vi "Aging Run.vi"(8 "UDL":path, 9 "error in":errorcluster, 10 "Arduino":refnum<visa-resource-name>, 11 "System Number":string) -> (1 "error out":errorcluster, 2 "Arduino":refnum<visa-resource-name>)   [LabVIEW 2024]
uses:
  <vilib>/addons/database/Connection.llb/DB Tools Open Connec (Path).vi
  <vilib>/addons/database/_DB Variant To Data/Database Variant To Data.xnode
  <vilib>/addons/database/NI_Database_API.lvlib
panel:
  out "Commands":string[](array[string])
  out "IsSine":bool=TRUE
  out "Frequency":string
  out "DC_SN":string
  out "Nominal Frequency":string
  out "OscVoltage":string
  out "TimeStart":string
  out "Current Position":i8
  out "Current Rack":i8
types:
  T1 = typedef "NI_Database_API.lvlib/Conn ObjectReference.ctl" = refnum<k1>
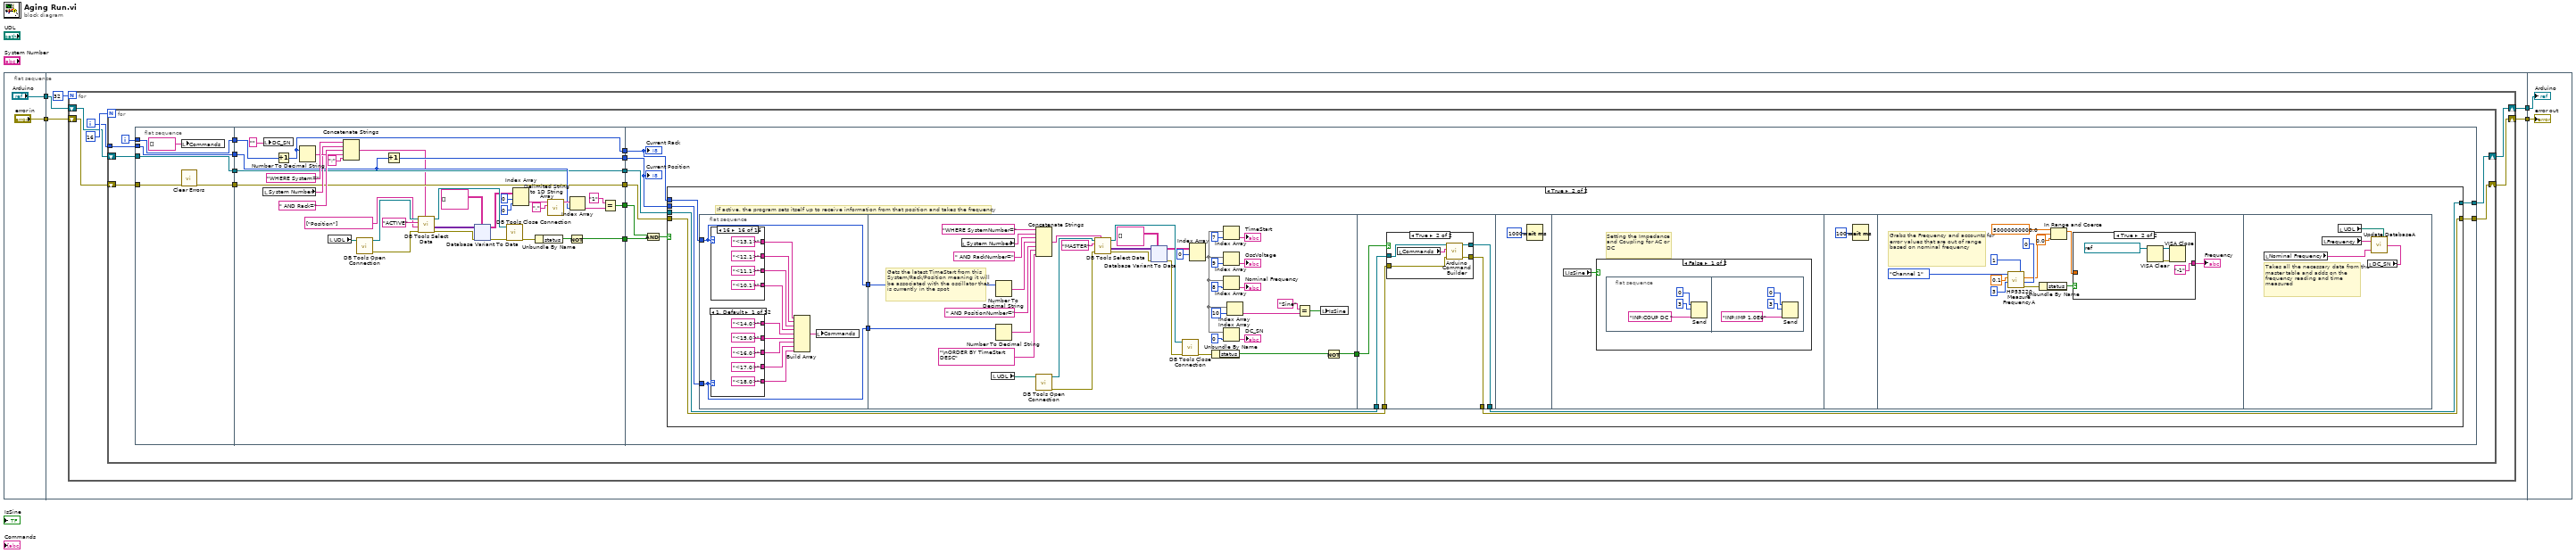
[diagram p0: block diagram]
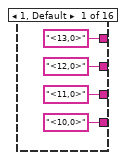
[diagram p3: hidden frame]
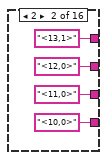
[diagram p4: hidden frame]
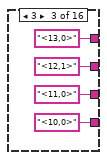
[diagram p5: hidden frame]
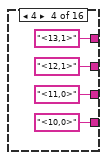
[diagram p6: hidden frame]
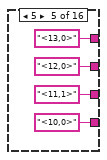
[diagram p7: hidden frame]
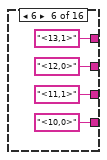
[diagram p8: hidden frame]
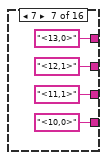
[diagram p9: hidden frame]
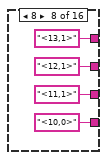
[diagram p10: hidden frame]
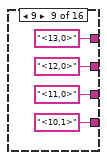
[diagram p11: hidden frame]
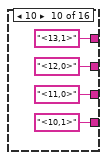
[diagram p12: hidden frame]
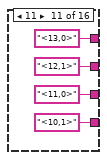
[diagram p13: hidden frame]
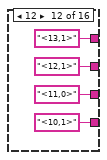
[diagram p14: hidden frame]
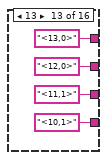
[diagram p15: hidden frame]
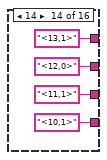
[diagram p16: hidden frame]
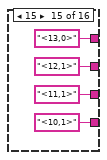
[diagram p17: hidden frame]
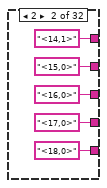
[diagram p18: hidden frame]
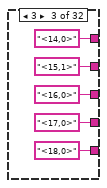
[diagram p19: hidden frame]
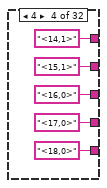
[diagram p20: hidden frame]
diagram:
  n1 = flat-sequence {
    tunnel: ["Arduino"] -> w2
    tunnel: ["error in"] -> w1
    tunnel: [w10] -> w4
    tunnel: [w9] -> w3
    tunnel: w2 -> [w8]
    tunnel: w1 -> [w7]
    tunnel: w4 -> [w507]
    tunnel: w3 -> [w506]
    frame #0 {
    }
    frame #1 {
      n2 = for {
        N: 32 -> [_]
        shift-right: [w15] -> w10
        shift-left: w8 -> [w13]
        shift-right: [w14] -> w9
        shift-left: w7 -> [w12]
        i -> [w16]
        n3 = for {
          N: 16 -> [_]
          tunnel: w16 -> [w31]
          shift-right: [w33] -> w14
          shift-left: w12 -> [w24]
          shift-right: [w32] -> w15
          shift-left: w13 -> [w23]
          i -> [w30]
          n4 = flat-sequence {
            tunnel: w30 -> [w38]
            tunnel: w31 -> [w39]
            tunnel: [w39] -> w26
            tunnel: [w38] -> w25
            tunnel: w24 -> [w37]
            tunnel: w23 -> [w35]
            tunnel: [w35] -> w20
            tunnel: [w34] -> w18
            tunnel: [w59] -> w29
            tunnel: [w58] -> w28
            tunnel: [w57] -> w27
            tunnel: w26 -> [w61]
            tunnel: w25 -> [w60]
            tunnel: [w55] -> w22
            tunnel: [w54] -> w21
            tunnel: w20 -> [w54]
            tunnel: [w53] -> w19
            tunnel: w18 -> [w53]
            tunnel: [w127] -> w33
            tunnel: [w126] -> w32
            tunnel: w29 -> [w123]
            tunnel: w28 -> [w124]
            tunnel: w27 -> [w125]
            tunnel: w22 -> [w122]
            tunnel: w21 -> [w120]
            tunnel: w19 -> [w119]
            frame #0 {
              n5 = local write "Commands"(string[] [] ("Commands")) -> ()
              n6 = call <vilib>:"Clear Errors.vi"("error in (no error)"=w37) -> ("error out"=w34:errorcluster)  [unwired: 5 in, 1 out]
            }
            frame #1 {
              n7 = local read "System Number"() -> (w70:string)
              n8 = local write "DC_SN"("" ("DC.SN")) -> ()
              n9 = Increment(x=w60) -> (x+1=w58:i32)
              n10 = Number To Decimal String(number=w58) -> (decimal integer string=w71:string)  [unwired: 1 in]
              n11 = local read "UDL"() -> (w44:path)
              n12 = Concatenate Strings("WHERE System=" ("SQL Query"), w70, " AND Rack=", w71, ";" ("string")) -> (w46:string)
              n13 = call-poly <vilib>:"DB Tools Open Connection.vi"("connection information"=w44) -> ("error out"=w50:errorcluster, "connection reference"=w51:T1)  [unwired: 7 in]
              n14 = Increment(x=w61) -> (x+1=w57:i32)
              n15 = call <vilib>:"DB Tools Select Data.vi"("condition"=w46, "error in (no error)"=w50, "columns"=string[] ["Position"], "table"="ACTIVE", "connection reference"=w51) -> ("error out"=w43:errorcluster, "data"=w48:variant[][], "connection reference out"=w52:T1)  [unwired: 1 in]
              n16 = xnode "Database Variant To Data"("database variant"=w48, "error in (no error)"=w43, "type"=string[][] [] ("table")) -> ("data"=w45:string[][], "error out"=w41:errorcluster)
              n17 = call <vilib>:"DB Tools Close Connection.vi"("error in (no error)"=w41, "connection reference"=w52) -> ("error out"=w42:errorcluster)  [unwired: 5 in]
              n18 = Index Array(array=w45, index (row)=0 ("disabled index (row)"), index (col)=0 ("disabled index (col)")) -> (element=w69:string)
              n19 = Unbundle By Name(w42) -> ("status"=w56:bool)
              n20 = call <vilib>:"Delimited String to 1D String Array.vi"("delimiter"=",", "delimited string"=w69) -> ("string array"=w66:string[])  [unwired: 9 in]
              n21 = Not(x=w56) -> (.not. x?=w55:bool)
              n22 = Index Array(array=w66, index=w61) -> (element=w65:string)
              n23 = Equal?(x="1", y=w65) -> (x = y?=w59:bool)
            }
            frame #2 {
              n24 = And(x=w123, y=w122) -> (x .and. y?=w121:bool)
              n25 = case shown="True" w121 {
                tunnel: w125 -> [_ w138]
                tunnel: w124 -> [_ w137]
                tunnel: [w128 w136] -> w127
                tunnel: [w129 w135] -> w126
                tunnel: w119 -> [w128 w134]
                tunnel: w120 -> [w129 w133]
                frame False {
                  # "If inactive, nothing happens"
                }
                frame True {
                  # "If active, the program sets itself up to receive information from that position and takes the frequency"
                  n26 = flat-sequence {
                    tunnel: [w150] -> w132
                    tunnel: [w149] -> w131
                    tunnel: w137 -> [w149]
                    tunnel: w138 -> [w150]
                    tunnel: w131 -> [w402]
                    tunnel: w132 -> [w404]
                    tunnel: [w387] -> w130
                    tunnel: [w460] -> w136
                    tunnel: [w459] -> w135
                    tunnel: w134 -> [w458]
                    tunnel: w133 -> [w457]
                    tunnel: w130 -> [w456]
                    frame #0 {
                      n27 = case shown="16" w149 {
                        tunnel: ["<10,0>" ("string") "<10,0>" ("string") "<10,0>" ("string") "<10,0>" ("string") "<10,0>" ("string") "<10,0>" ("string") "<10,0>" ("string") "<10,0>" ("string") "<10,1>" ("string") "<10,1>" ("string") "<10,1>" ("string") "<10,1>" ("string") "<10,1>" ("string") "<10,1>" ("string") "<10,1>" ("string") "<10,1>" ("string")] -> w146
                        tunnel: ["<12,0>" ("string") "<12,0>" ("string") "<12,1>" ("string") "<12,1>" ("string") "<12,0>" ("string") "<12,0>" ("string") "<12,1>" ("string") "<12,1>" ("string") "<12,0>" ("string") "<12,0>" ("string") "<12,1>" ("string") "<12,1>" ("string") "<12,0>" ("string") "<12,0>" ("string") "<12,1>" ("string") "<12,1>" ("string")] -> w147
                        tunnel: ["<11,0>" ("string") "<11,0>" ("string") "<11,0>" ("string") "<11,0>" ("string") "<11,1>" ("string") "<11,1>" ("string") "<11,1>" ("string") "<11,1>" ("string") "<11,0>" ("string") "<11,0>" ("string") "<11,0>" ("string") "<11,0>" ("string") "<11,1>" ("string") "<11,1>" ("string") "<11,1>" ("string") "<11,1>" ("string")] -> w148
                        tunnel: ["<13,0>" ("string") "<13,1>" ("string") "<13,0>" ("string") "<13,1>" ("string") "<13,0>" ("string") "<13,1>" ("string") "<13,0>" ("string") "<13,1>" ("string") "<13,0>" ("string") "<13,1>" ("string") "<13,0>" ("string") "<13,1>" ("string") "<13,0>" ("string") "<13,1>" ("string") "<13,0>" ("string") "<13,1>" ("string")] -> w145
                        frame 1, Default {
                        }
                        frame 2 {
                        }
                        frame 3 {
                        }
                        frame 4 {
                        }
                        frame 5 {
                        }
                        frame 6 {
                        }
                        frame 7 {
                        }
                        frame 8 {
                        }
                        frame 9 {
                        }
                        frame 10 {
                        }
                        frame 11 {
                        }
                        frame 12 {
                        }
                        frame 13 {
                        }
                        frame 14 {
                        }
                        frame 15 {
                        }
                        frame 16 {
                        }
                      }
                      n28 = case shown="1, Default" w150 {
                        tunnel: ["<14,0>" ("string") "<14,1>" ("string") "<14,0>" ("string") "<14,1>" ("string") "<14,0>" ("string") "<14,1>" ("string") "<14,0>" ("string") "<14,1>" ("string") "<14,0>" ("string") "<14,1>" ("string") "<14,0>" ("string") "<14,1>" ("string") "<14,0>" ("string") "<14,1>" ("string") "<14,0>" ("string") "<14,1>" ("string") "<14,0>" ("string") "<14,1>" ("string") "<14,0>" ("string") "<14,1>" ("string") "<14,0>" ("string") "<14,1>" ("string") "<14,0>" ("string") "<14,1>" ("string") "<14,0>" ("string") "<14,1>" ("string") "<14,0>" ("string") "<14,1>" ("string") "<14,0>" ("string") "<14,1>" ("string") "<14,0>" ("string") "<14,1>" ("string")] -> w143
                        tunnel: ["<16,0>" ("string") "<16,0>" ("string") "<16,0>" ("string") "<16,0>" ("string") "<16,1>" ("string") "<16,1>" ("string") "<16,1>" ("string") "<16,1>" ("string") "<16,0>" ("string") "<16,0>" ("string") "<16,0>" ("string") "<16,0>" ("string") "<16,1>" ("string") "<16,1>" ("string") "<16,1>" ("string") "<16,1>" ("string") "<16,0>" ("string") "<16,0>" ("string") "<16,0>" ("string") "<16,0>" ("string") "<16,1>" ("string") "<16,1>" ("string") "<16,1>" ("string") "<16,1>" ("string") "<16,0>" ("string") "<16,0>" ("string") "<16,0>" ("string") "<16,0>" ("string") "<16,1>" ("string") "<16,1>" ("string") "<16,1>" ("string") "<16,1>" ("string")] -> w141
                        tunnel: ["<18,0>" ("string") "<18,0>" ("string") "<18,0>" ("string") "<18,0>" ("string") "<18,0>" ("string") "<18,0>" ("string") "<18,0>" ("string") "<18,0>" ("string") "<18,0>" ("string") "<18,0>" ("string") "<18,0>" ("string") "<18,0>" ("string") "<18,0>" ("string") "<18,0>" ("string") "<18,0>" ("string") "<18,0>" ("string") "<18,1>" ("string") "<18,1>" ("string") "<18,1>" ("string") "<18,1>" ("string") "<18,1>" ("string") "<18,1>" ("string") "<18,1>" ("string") "<18,1>" ("string") "<18,1>" ("string") "<18,1>" ("string") "<18,1>" ("string") "<18,1>" ("string") "<18,1>" ("string") "<18,1>" ("string") "<18,1>" ("string") "<18,1>" ("string")] -> w139
                        tunnel: ["<15,0>" ("string") "<15,0>" ("string") "<15,1>" ("string") "<15,1>" ("string") "<15,0>" ("string") "<15,0>" ("string") "<15,1>" ("string") "<15,1>" ("string") "<15,0>" ("string") "<15,0>" ("string") "<15,1>" ("string") "<15,1>" ("string") "<15,0>" ("string") "<15,0>" ("string") "<15,1>" ("string") "<15,1>" ("string") "<15,0>" ("string") "<15,0>" ("string") "<15,1>" ("string") "<15,1>" ("string") "<15,0>" ("string") "<15,0>" ("string") "<15,1>" ("string") "<15,1>" ("string") "<15,0>" ("string") "<15,0>" ("string") "<15,1>" ("string") "<15,1>" ("string") "<15,0>" ("string") "<15,0>" ("string") "<15,1>" ("string") "<15,1>" ("string")] -> w142
                        tunnel: ["<17,0>" ("string") "<17,0>" ("string") "<17,0>" ("string") "<17,0>" ("string") "<17,0>" ("string") "<17,0>" ("string") "<17,0>" ("string") "<17,0>" ("string") "<17,1>" ("string") "<17,1>" ("string") "<17,1>" ("string") "<17,1>" ("string") "<17,1>" ("string") "<17,1>" ("string") "<17,1>" ("string") "<17,1>" ("string") "<17,0>" ("string") "<17,0>" ("string") "<17,0>" ("string") "<17,0>" ("string") "<17,0>" ("string") "<17,0>" ("string") "<17,0>" ("string") "<17,0>" ("string") "<17,1>" ("string") "<17,1>" ("string") "<17,1>" ("string") "<17,1>" ("string") "<17,1>" ("string") "<17,1>" ("string") "<17,1>" ("string") "<17,1>" ("string")] -> w140
                        frame 1, Default {
                        }
                        frame 2 {
                        }
                        frame 3 {
                        }
                        frame 4 {
                        }
                        frame 5 {
                        }
                        frame 6 {
                        }
                        frame 7 {
                        }
                        frame 8 {
                        }
                        frame 9 {
                        }
                        frame 10 {
                        }
                        frame 11 {
                        }
                        frame 12 {
                        }
                        frame 13 {
                        }
                        frame 14 {
                        }
                        frame 15 {
                        }
                        frame 16 {
                        }
                        frame 17 {
                        }
                        frame 18 {
                        }
                        frame 19 {
                        }
                        frame 20 {
                        }
                        frame 21 {
                        }
                        frame 22 {
                        }
                        frame 23 {
                        }
                        frame 24 {
                        }
                        frame 25 {
                        }
                        frame 26 {
                        }
                        frame 27 {
                        }
                        frame 28 {
                        }
                        frame 29 {
                        }
                        frame 30 {
                        }
                        frame 31 {
                        }
                        frame 32 {
                        }
                      }
                      n29 = Build Array(w145, w147, w148, w146, w143, w142, w141, w140, w139) -> (w144:string[])
                      n30 = local write "Commands"(w144) -> ()
                    }
                    frame #1 {
                      # "Gets the latest TimeStart from this System/Rack/Position meaning it will be associated with the oscillator that is currently in the spot"
                      n31 = local read "System Number"() -> (w411:string)
                      n32 = local read "UDL"() -> (w378:path)
                      n33 = Number To Decimal String(number=w402) -> (decimal integer string=w409:string)  [unwired: 1 in]
                      n34 = Number To Decimal String(number=w404) -> (decimal integer string=w410:string)  [unwired: 1 in]
                      n35 = Concatenate Strings("WHERE SystemNumber=" ("SQL Query"), w411, " AND RackNumber=" ("string"), w409, " AND PositionNumber=" ("string"), w410, "\nORDER BY TimeStart DESC" ("string")) -> (w380:string)
                      n36 = call-poly <vilib>:"DB Tools Open Connection.vi"("connection information"=w378) -> ("error out"=w384:errorcluster, "connection reference"=w385:T1)  [unwired: 7 in]
                      n37 = call <vilib>:"DB Tools Select Data.vi"("condition"=w380, "error in (no error)"=w384, "table"="MASTER", "connection reference"=w385) -> ("error out"=w376:errorcluster, "data"=w382:variant[][], "connection reference out"=w386:T1)  [unwired: 2 in]
                      n38 = xnode "Database Variant To Data"("database variant"=w382, "error in (no error)"=w376, "type"=string[][] [] ("table")) -> ("data"=w377:string[][], "error out"=w375:errorcluster)
                      n39 = call <vilib>:"DB Tools Close Connection.vi"("error in (no error)"=w375, "connection reference"=w386) -> ("error out"=w379:errorcluster)  [unwired: 5 in]
                      n40 = Index Array(array=w377, index (row)=0 ("disabled index (row)")) -> (element=w389:string[])  [unwired: 1 in]
                      n41 = Unbundle By Name(w379) -> ("status"=w388:bool)
                      n42 = Index Array(array=w389, index=7) -> (element=→"TimeStart":string)
                      n43 = Index Array(array=w389, index=9) -> (element=→"OscVoltage":string)
                      n44 = Index Array(array=w389, index=8) -> (element=→"Nominal Frequency":string)
                      n45 = Index Array(array=w389, index=0) -> (element=→"DC_SN":string)
                      n46 = Index Array(array=w389, index=10) -> (element=w399:string)
                      n47 = Equal?(x="Sine", y=w399) -> (x = y?=w400:bool)
                      n48 = local write "IsSine"(w400) -> ()
                      n49 = Not(x=w388) -> (.not. x?=w387:bool)
                    }
                    frame #2 {
                      n50 = case shown="True" w456 {
                        tunnel: [w461 w467] -> w460
                        tunnel: [w462 w466] -> w459
                        tunnel: w458 -> [w461 w465]
                        tunnel: w457 -> [w462 w464]
                        frame False {
                        }
                        frame True {
                          n51 = local read "Commands"() -> (w463:string[])
                          n52 = call "Arduino Command Builder.vi"("error in"=w465, "Commands"=w463, "Arduino in"=w464) -> ("error out"=w467:errorcluster, "Arduino out"=w466:refnum<visa-resource-name>)  [unwired: 7 in]
                        }
                      }
                    }
                    frame #3 {
                      n53 = Wait (ms)(milliseconds to wait=u32 1000 ("millisecond multiple")) -> ()  [unwired: 1 out]
                    }
                    frame #4 {
                      # "Setting the Impedance and Coupling for AC or DC"
                      n54 = local read "IsSine"() -> (w469:bool)
                      n55 = case shown="False" w469 {
                        frame False {
                          n56 = flat-sequence {
                            frame #0 {
                              n57 = Send(0:0 ("bus"), 2:i16 3 ("address"), 5:"INP:COUP DC " ("data string")) -> ()  [unwired: 2 in, 3 out]
                            }
                            frame #1 {
                              n58 = Send(0:0 ("bus"), 2:i16 3 ("address"), 5:"INP:IMP 1.0E6" ("data string")) -> ()  [unwired: 2 in, 3 out]
                            }
                          }
                        }
                        frame True {
                          n59 = flat-sequence {
                            frame #0 {
                              n60 = Send(0:0 ("bus"), 2:i16 3 ("address"), 5:"INP:COUP AC " ("data string")) -> ()  [unwired: 2 in, 3 out]
                            }
                            frame #1 {
                              n61 = Send(0:0 ("bus"), 2:i16 3 ("address"), 5:"INP:IMP 50" ("data string")) -> ()  [unwired: 2 in, 3 out]
                            }
                          }
                        }
                      }
                    }
                    frame #5 {
                      n62 = Wait (ms)(milliseconds to wait=u32 100 ("millisecond multiple")) -> ()  [unwired: 1 out]
                    }
                    frame #6 {
                      # "Grabs the Frequency and accounts for error values that are out of range based on nominal frequency"
                      n63 = call "HP53220 Measure FrequencyA.vi"("GPIB Bus"=0, "Number of Readings"=1, "GPIB Address"=i16 3, "Gate Time"=0.1, "Channel(1,2,3)"=enum16{"Channel 1", "Channel 2", "Channel 3"}."Channel 1") -> ("error out"=w489:errorcluster, "Frequency"=w490:dbl)  [unwired: 1 in]
                      n64 = Unbundle By Name(w489) -> ("status"=w488:bool)
                      n65 = In Range and Coerce(upper limit=50000000000.0 ("y"), x=w490, lower limit=0.0) -> (coerced(x)=w487:dbl)  [unwired: 1 out]
                      n66 = case shown="True" w488 {
                        tunnel: w487 -> [w496 _]
                        tunnel: [w495 "-1"] -> w486
                        frame False {
                          n67 = Format Into String(format string="%.6f", w496) -> (resulting string=w495:string)  [unwired: 2 in, 1 out]
                        }
                        frame True {
                          n68 = VISA Clear(VISA resource name=refnum<visa-resource-name> "GPIB0::3::INSTR") -> (VISA resource name out=w499:refnum<visa-resource-name>, error out=w498:errorcluster)  [unwired: 1 in]
                          n69 = VISA Close(VISA resource name=w499, error in (no error)=w498) -> ()  [unwired: 1 out]
                        }
                      }
                      "Frequency" <- w486
                    }
                    frame #7 {
                      # "Takes all the necessary data from the master table and adds on the frequency reading and time measured"
                      n70 = local read "Nominal Frequency"() -> (w504:string)
                      n71 = local read "Frequency"() -> (w505:string)
                      n72 = local read "UDL"() -> (w502:path)
                      n73 = local read "DC_SN"() -> (w503:string)
                      n74 = call "Update DatabaseA.vi"("Frequency"=w505, "Nominal Frequency"=w504, "connection information"=w502, "DC_SN"=w503) -> ()  [unwired: 1 in]
                    }
                  }
                }
              }
              "Current Rack" <- w124
              "Current Position" <- w125
            }
          }
        }
      }
    }
    frame #2 {
      "Arduino" <- w507
      "error out" <- w506
    }
  }
